vi "Receiver UI.vi"(8 "Error In":errorcluster) -> (0 "Error Out":errorcluster, 3 "Message":variant)   [LabVIEW 2023, in "User Receiver.lvclass"]
uses:
  User Receiver.lvclass
  Controls/Queue Operation.ctl
  Controls/Receiver Data.ctl
  Controls/User Event Operations.ctl
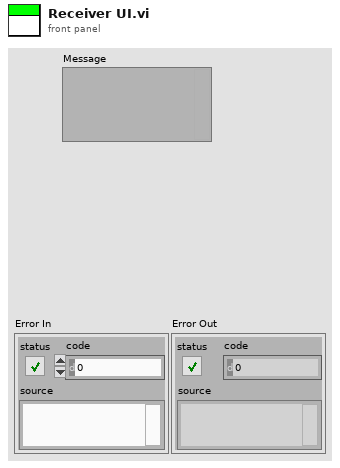
[diagram p1: front panel]
types:
  T1 = typedef "User Event Operations.ctl" = enum16{"Obtain", "Generate", "Destroy"}
  T2 = typedef "Receiver Data.ctl" = cluster{"Variant":variant}
  T3 = typedef "Queue Operation.ctl" = enum16{"Create & Enqueue N", "Enqueue N", "Dequeue", "Enstack N", "Flush", "Release"}
  T4 = typedef "Queue Element.ctl" = cluster{"State":string, "Data":variant}
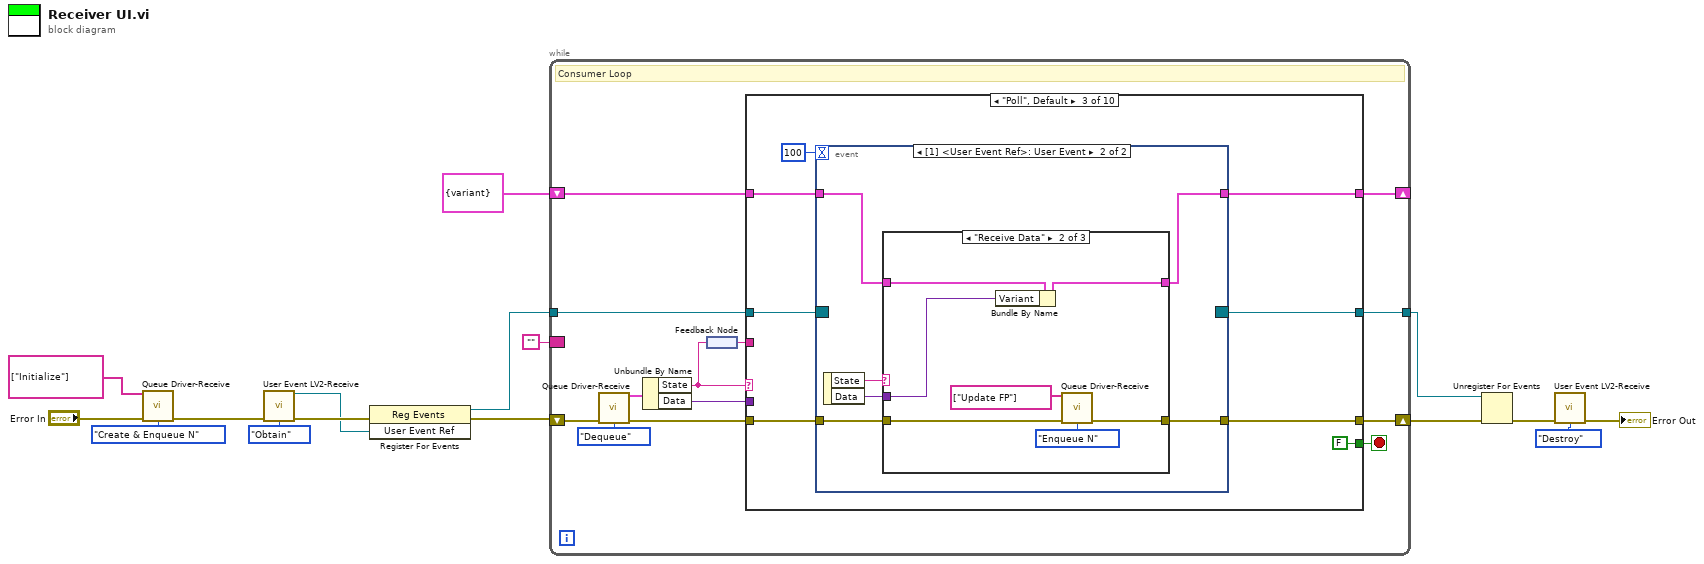
[diagram p0: block diagram]
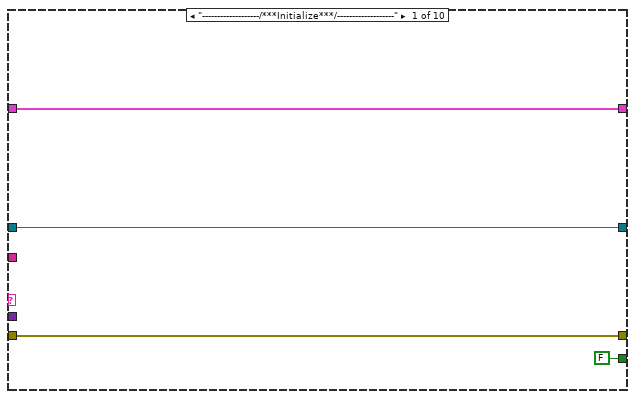
[diagram p2: hidden frame]
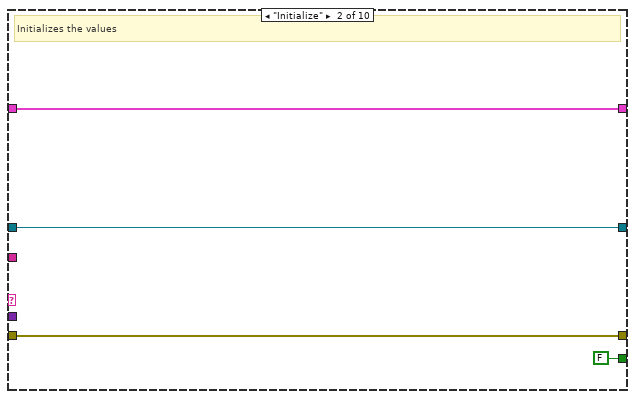
[diagram p3: hidden frame]
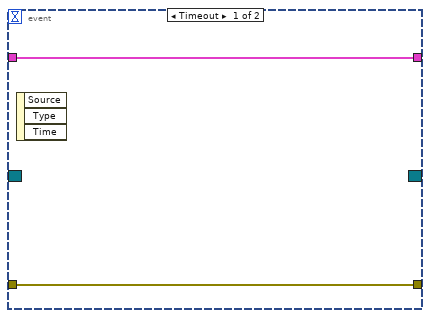
[diagram p4: hidden frame]
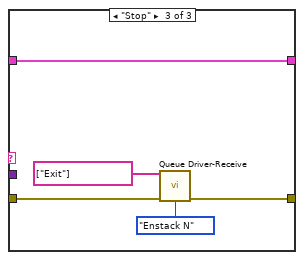
[diagram p6: hidden frame]
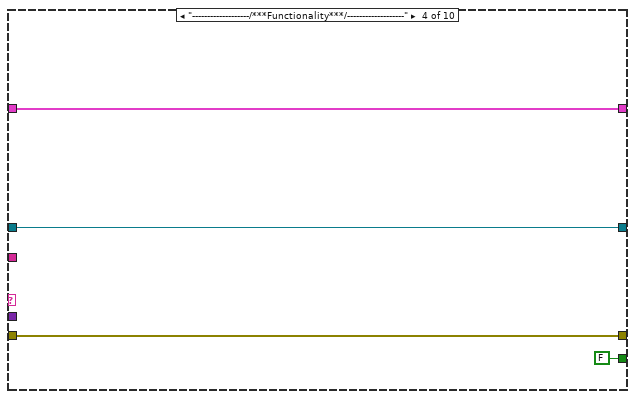
[diagram p7: hidden frame]
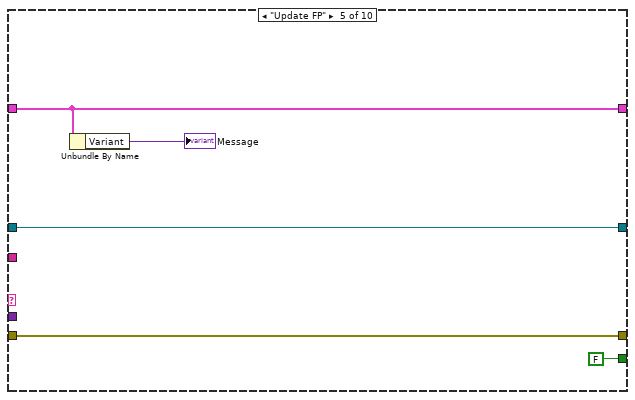
[diagram p8: hidden frame]
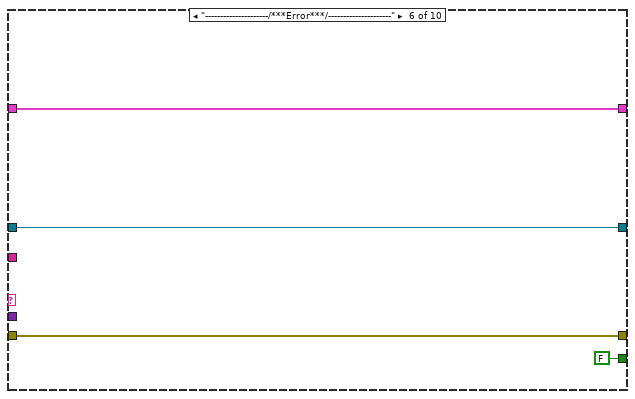
[diagram p9: hidden frame]
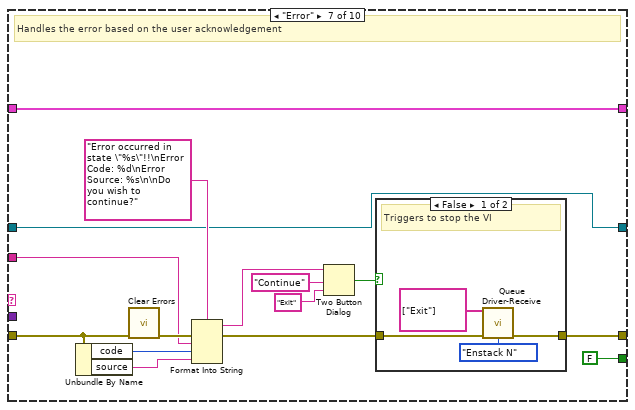
[diagram p10: hidden frame]
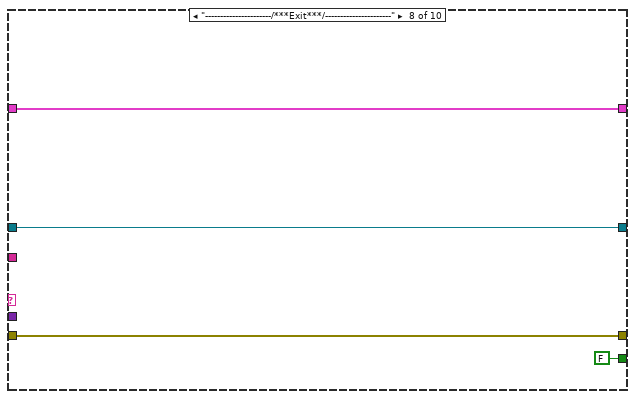
[diagram p12: hidden frame]
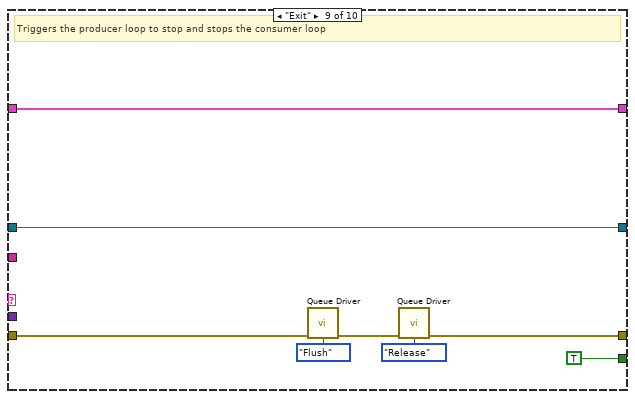
[diagram p13: hidden frame]
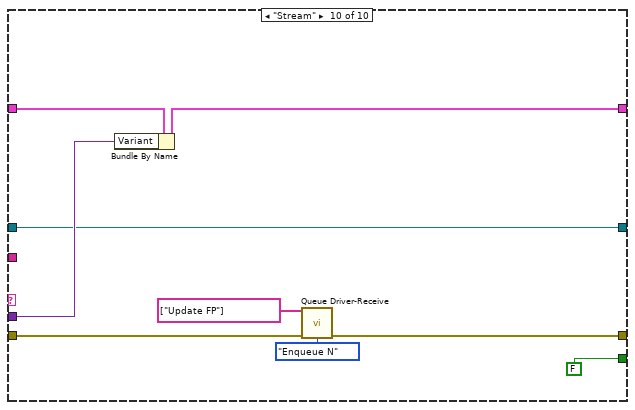
[diagram p14: hidden frame]
diagram:
  n1 = call "Queue Driver-Receive.vi"("States[]"=string[] ["Initialize"], "Error In"="Error In", "Queue Operation"=Queue_Operation."Create & Enqueue N") -> ("Error Out"=w13:errorcluster)  [unwired: 11 in, 1 out]
  n2 = call "User Event LV2-Receive.vi"("Error In"=w13, "Operation"=User_Event_Operations."Obtain") -> ("User Event Ref"=w6:refnum<user-event>, "Error Out"=w9:errorcluster)  [unwired: 12 in]
  n3 = register-events(error in=w9, w6) -> (reference out=w5:refnum<event-registration>, error out=w7:errorcluster)  [unwired: 1 in]
  n4 = while {
    shift-right: [w28] -> w14
    shift-left: w7 -> [w29]
    border: "" -> [_]
    shift-right: [w19] -> _
    shift-left: T2 {"Variant"=variant(dbl 0.0)} -> [w20]
    tunnel: w5 -> [w18]
    tunnel: [w17] -> w3
    stop <- w24 stop-if-true
    # "Consumer Loop"
    n5 = call "Queue Driver-Receive.vi"("Error In"=w29, "Queue Operation"=Queue_Operation."Dequeue") -> ("Dequeue Element"=w25:T4, "Error Out"=w27:errorcluster)  [unwired: 12 in]
    n6 = Unbundle By Name(w25) -> ("State"=w23:string, "Data"=w21:variant)
    n7 = feedback-in #1(w23) -> ()
    n8 = feedback #1() -> (w22:string)
    n9 = case shown="\"Poll\", Default" w23 {
      tunnel: w27 -> [w33 w36 w45 w71 w76 w80 w87 w104 w112 w121]
      tunnel: [w33 w36 w43 w71 w76 w80 w84 w104 w108 w115] -> w28
      tunnel: [FALSE FALSE FALSE FALSE FALSE FALSE FALSE FALSE TRUE FALSE] -> w24
      tunnel: w22 -> [_ _ _ _ _ _ w85 _ _ _]
      tunnel: w21 -> [_ _ _ _ _ _ _ _ _ w117]
      tunnel: w20 -> [w31 w35 w42 w69 w73 w78 w82 w102 w106 w120]
      tunnel: [w31 w35 w41 w69 w73 w78 w82 w102 w106 w118] -> w19
      tunnel: w18 -> [w30 w34 w39 w68 w74 w77 w81 w101 w105 w116]
      tunnel: [w30 w34 w38 w68 w74 w77 w81 w101 w105 w116] -> w17
      frame "-------------------/***Initialize***/-------------------" {
      }
      frame "Initialize" {
        # "Initializes the values"
      }
      frame "Poll", Default {
        n10 = event shown="[1] <User Event Ref>: User Event" {
          selector: w39 -> [_ _]
          dyn-events: [_ _] -> w38
          timeout: 100 -> [_ _]
          tunnel: w45 -> [w47 w53]
          tunnel: [w47 w52] -> w43
          tunnel: [w46 w48] -> w41
          tunnel: w42 -> [w46 w49]
          event Timeout {
            n11 = event-data() -> ()  [unwired: 1 in, 3 out]
          }
          event User Event {
            n12 = event-data() -> ("State"=w51:string, "Data"=w50:variant)  [unwired: 1 in]
            n13 = case shown="\"Receive Data\"" w51 {
              tunnel: w53 -> [w55 w62 w67]
              tunnel: [w55 w59 w65] -> w52
              tunnel: w50 -> [_ w56 _]
              tunnel: [w54 w60 w66] -> w48
              tunnel: w49 -> [w54 w61 w66]
              frame "False", Default {
              }
              frame "Receive Data" {
                n14 = Bundle By Name(cluster=w61, "Variant"=w56) -> (w60:T2)
                n15 = call "Queue Driver-Receive.vi"("States[]"=string[] ["Update FP"], "Error In"=w62, "Queue Operation"=Queue_Operation."Enqueue N") -> ("Error Out"=w59:errorcluster)  [unwired: 11 in, 1 out]
              }
              frame "Stop" {
                n16 = call "Queue Driver-Receive.vi"("States[]"=string[] ["Exit"], "Error In"=w67, "Queue Operation"=Queue_Operation."Enstack N") -> ("Error Out"=w65:errorcluster)  [unwired: 11 in, 1 out]
              }
            }
          }
        }
      }
      frame "-------------------/***Functionality***/-------------------" {
      }
      frame "Update FP" {
        n17 = Unbundle By Name(w73) -> ("Variant"=→"Message":variant)
      }
      frame "---------------------/***Error***/---------------------" {
      }
      frame "Error" {
        # "Handles the error based on the user acknowledgement"
        n18 = Unbundle By Name(w87) -> ("code"=w89:i32, "source"=w88:string)
        n19 = call <vilib>:"Clear Errors.vi"("error in (no error)"=w87) -> ("error out"=w94:errorcluster)  [unwired: 5 in, 1 out]
        n20 = Format Into String(format string="Error occurred in state \"%s\"!!\nError Code: %d\nError Source: %s\n\nDo you wish to continue?", error in=w94, w85, w89, w88) -> (resulting string=w92:string, error out=w86:errorcluster)  [unwired: 1 in]
        n21 = Two Button Dialog(message=w92, 1:"Exit" ("F button name (\"Cancel\")"), 2:"Continue" ("T button name (\"OK\")")) -> (T button?=w83:bool)
        n22 = case shown="False" w83 {
          tunnel: w86 -> [w99 w100]
          tunnel: [w98 w100] -> w84
          frame False {
            # "Triggers to stop the VI"
            n23 = call "Queue Driver-Receive.vi"("States[]"=string[] ["Exit"], "Error In"=w99, "Queue Operation"=Queue_Operation."Enstack N") -> ("Error Out"=w98:errorcluster)  [unwired: 11 in, 1 out]
          }
          frame True {
          }
        }
      }
      frame "----------------------/***Exit***/----------------------" {
      }
      frame "Exit" {
        # "Triggers the producer loop to stop and stops the consumer loop"
        n24 = call "Queue Driver.vi"("Error In"=w112, "Queue Operation"=Queue_Operation."Flush") -> ("Error Out"=w110:errorcluster)  [unwired: 12 in, 1 out]
        n25 = call "Queue Driver.vi"("Error In"=w110, "Queue Operation"=Queue_Operation."Release") -> ("Error Out"=w108:errorcluster)  [unwired: 12 in, 1 out]
      }
      frame "Stream" {
        n26 = Bundle By Name(cluster=w120, "Variant"=w117) -> (w118:T2)
        n27 = call "Queue Driver-Receive.vi"("States[]"=string[] ["Update FP"], "Error In"=w121, "Queue Operation"=Queue_Operation."Enqueue N") -> ("Error Out"=w115:errorcluster)  [unwired: 11 in, 1 out]
      }
    }
  }
  n28 = Unregister For Events(event registration refnum=w3, error in=w14) -> (error out=w4:errorcluster)
  n29 = call "User Event LV2-Receive.vi"("Error In"=w4, "Operation"=User_Event_Operations."Destroy") -> ("Error Out"=→"Error Out":errorcluster)  [unwired: 12 in, 1 out]
